vi "Get TestPN.vi"(8 "error in (no error)":errorcluster, 11 "niDTS WLAN DUT in":refnum<class "niDTS WLAN Dut.lvclass">) -> (0 "error out":errorcluster, 2 "String":string, 3 "niDTS WLAN DUT out":refnum<class "niDTS WLAN Dut.lvclass">)   [LabVIEW 2015, in "niDTS WLAN.lvlib" / "niDTS WLAN Dut.lvclass"]
uses:
  niDTS WLAN Dut.lvclass
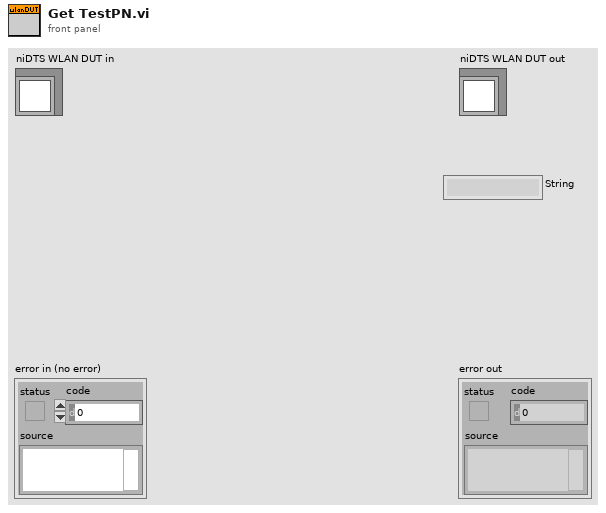
[diagram p1: front panel]
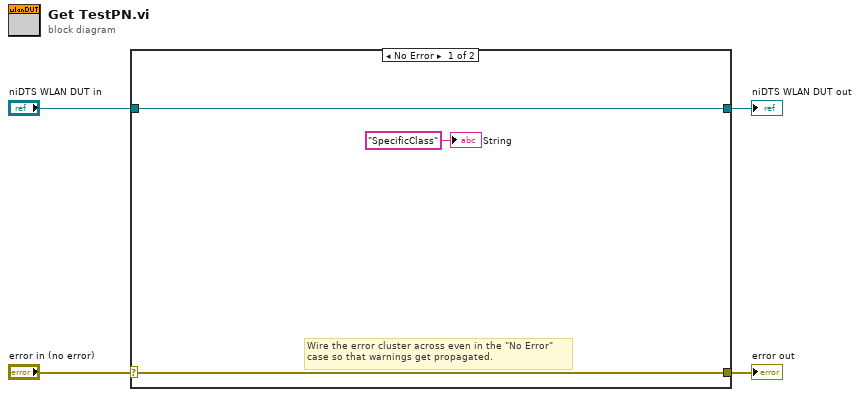
[diagram p0: block diagram]
diagram:
  n1 = case shown="No Error" "error in (no error)" {
    selector: "error in (no error)" -> [w6 w9]
    tunnel: [w6 w9] -> w3
    tunnel: [w7 w8] -> w1
    tunnel: "niDTS WLAN DUT in" -> [w7 w8]
    frame No Error {
      # "Wire the error cluster across even in the \"No Error\"\ncase so that warnings get propagated."
      "String" <- "SpecificClass" ("String")
    }
    frame Error {
    }
  }
  "error out" <- w3
  "niDTS WLAN DUT out" <- w1
